vi "Wait till motion stops.vi"(8 "error in":errorcluster, 9 "Timeout (sec)":dbl=100.0, 10 "Index":i32, 11 "Visa Array Out":refnum<visa-resource-name>[](array[refnum])) -> (0 "error out":errorcluster, 1 "Time out?":bool, 2 "Current Posistion":dbl, 3 "Visa array out":refnum<visa-resource-name>[](array[refnum]))   [LabVIEW 2010, in "SignalWriterMH110203USBStepperMotor.lvclass"]
uses:
  SignalWriterMH110203USBStepperMotor.lvclass
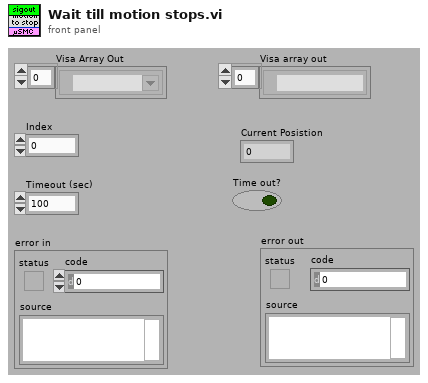
[diagram p1: front panel]
types:
  T1 = typedef "SignalWriterMH110203USBStepperMotor.lvclass/Get State Control (uSMC).ctl" = cluster{"Current Posistion":dbl, "CW/CCW":bool, "Speed":u16, "Temperature":dbl, "Power":u16, "Limit Switch 1":bool, "Limit Switch 2":bool, "After Reset":bool, "Step":u8, "Backlash":bool, "RT Error":bool, "RT State":bool, "Sync In":bool, "Sync Out":bool, "Ext Disconnect":bool, "Usb Powered":bool, "Voltage":dbl, "Working":bool, "SM Position in Encoder Units":i32, "Encoder Current Position":i32}
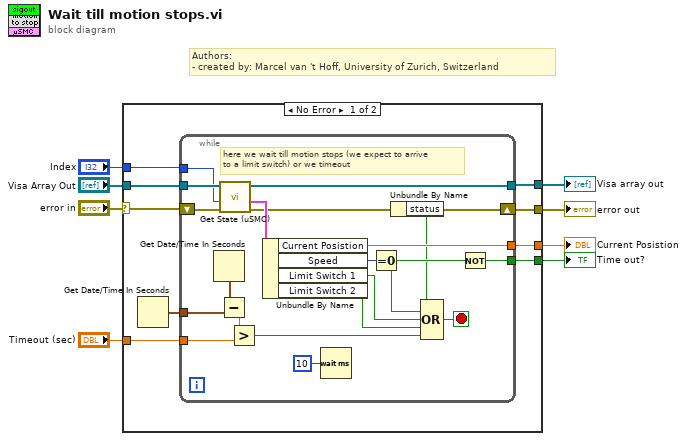
[diagram p0: block diagram]
diagram:
  # "Authors: \n- created by: Marcel van 't Hoff, University of Zurich, Switzerland"
  n1 = case shown="No Error" "error in" {
    selector: "error in" -> [w9 w38]
    tunnel: [w17 _] -> w8
    tunnel: "Index" -> [w16 _]
    tunnel: "Timeout (sec)" -> [w15 _]
    tunnel: [w13 w38] -> w5
    tunnel: [w12 w39] -> w4
    tunnel: "Visa Array Out" -> [w11 w39]
    tunnel: [w10 _] -> w2
    frame No Error {
      n2 = Get Date/Time In Seconds() -> (seconds since 1Jan1904=w14:timestamp)
      n3 = while {
        shift-right: [w22] -> w13
        shift-left: w9 -> [w37]
        tunnel: w11 -> [w36]
        tunnel: w16 -> [w21]
        tunnel: [w33] -> w12
        tunnel: w14 -> [w31]
        tunnel: w15 -> [w29]
        tunnel: [w28] -> w17
        tunnel: [w27] -> w10
        stop <- w23 stop-if-true
        # "here we wait till motion stops (we expect to arrive\nto a limit switch) or we timeout"
        n4 = Get Date/Time In Seconds() -> (seconds since 1Jan1904=w32:timestamp)
        n5 = Subtract(x=w32, y=w31) -> (x-y=w30:dbl)
        n6 = call "Get State (uSMC).vi"("error in (no error)"=w37, "SM number"=w21, "Visa array in"=w36) -> ("error out"=w22:errorcluster, "State cluster"=w35:T1, "Visa array out"=w33:refnum<visa-resource-name>[])  [unwired: 6 in]
        n7 = Greater?(x=w30, y=w29) -> (0:w24:bool)
        n8 = Unbundle By Name(w35) -> ("Current Posistion"=w27:dbl, "Speed"=w34:u16, "Limit Switch 1"=w26:bool, "Limit Switch 2"=w25:bool)
        n9 = Wait (ms)(milliseconds to wait=u32 10) -> ()  [unwired: 1 out]
        n10 = Equal To 0?(x=w34) -> (x = 0?=w20:bool)
        n11 = Unbundle By Name(w22) -> ("status"=w19:bool)
        n12 = Compound Arithmetic op=OR(w19, w20, w26, w25, w24) -> (w23:bool)
        n13 = Not(x=w20) -> (.not. x?=w28:bool)
      }
    }
    frame Error {
    }
  }
  "Time out?" <- w8
  "error out" <- w5
  "Visa array out" <- w4
  "Current Posistion" <- w2
